vi "PQgetColumn.vi"(8 "error in":errorcluster, 10 "query":string, 11 "conn":u32) -> (0 "error out":errorcluster, 2 "Data":string[](array[string]), 3 "conn_out":u32)   [LabVIEW 2019, in "libpqutility.lvlib"]
uses:
  libpqutility.lvlib
  libpqlv/src/PQgetvalue.vi
  libpqlv/src/PQntuples.vi
  libpqlv/libpqlv.lvlib
panel:
  out "PQsendQuery":i32
  out "PQresultStatus":T1(ring)
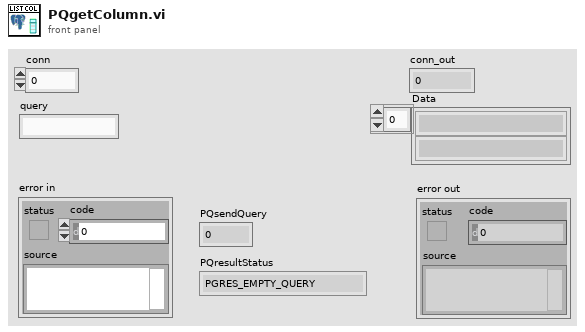
[diagram p1: front panel]
types:
  T1 = enum32{"PGRES_EMPTY_QUERY", "PGRES_COMMAND_OK", "PGRES_TUPLES_OK", "PGRES_COPY_OUT", "PGRES_COPY_IN", "PGRES_BAD_RESPONSE", "PGRES_NONFATAL_ERROR", "PGRES_FATAL_ERROR"}
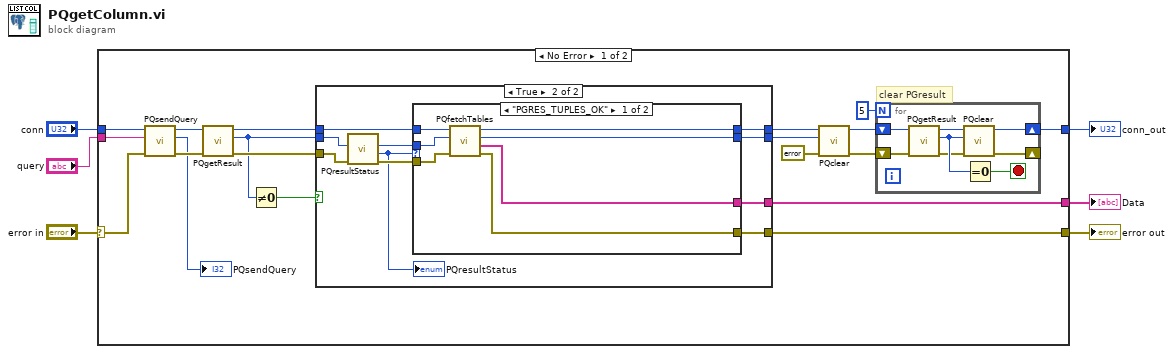
[diagram p0: block diagram]
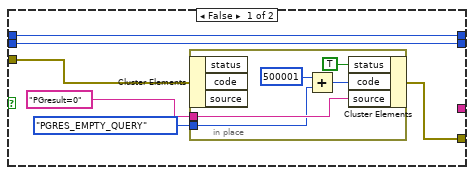
[diagram p2: hidden frame]
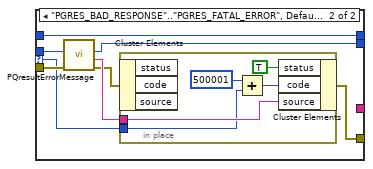
[diagram p3: hidden frame]
diagram:
  n1 = case shown="No Error" "error in" {
    selector: "error in" -> [w16 w76]
    tunnel: "conn" -> [w17 w75]
    tunnel: [w18 w76] -> w5
    tunnel: [w9 w75] -> w3
    tunnel: [w15 _] -> w2
    tunnel: "query" -> [w10 _]
    frame No Error {
      # "clear PGresult"
      n2 = call "PQsendQuery.vi"("error in (no error)"=w16, "query"=w10, "conn"=w17) -> ("error out"=w25:errorcluster, "PQsendQuery"=→"PQsendQuery":i32, "conn_out"=w14:u32)  [unwired: 6 in]
      n3 = call "PQgetResult.vi"("error in (no error)"=w25, "conn"=w14) -> ("error out"=w24:errorcluster, "PGresult"=w23:u32, "conn_out"=w13:u32)  [unwired: 7 in]
      n4 = Not Equal To 0?(x=w23) -> (x != 0?=w22:bool)
      n5 = case shown="True" w22 {
        tunnel: w24 -> [w28 w46]
        tunnel: w13 -> [w30 w45]
        tunnel: [_ w43] -> w15
        tunnel: [w27 w42] -> w18
        tunnel: w23 -> [w31 w41]
        tunnel: [w31 w39] -> w19
        tunnel: [w30 w37] -> w12
        frame False {
          n6 = in-place {
            in-place-border: "PGresult=0" ("source") -> [w36]
            in-place-border: T1."PGRES_EMPTY_QUERY" ("PQresultStatus") -> [w33]
            n7 = in-place-cluster #1(w28) -> ()  [unwired: 3 out]
            n8 = Add(x=u32 500001, y=w33) -> (x+y=w32:u32)
            n9 = in-place-cluster #1("status"=TRUE, "code"=w32, "source"=w36) -> (w27:errorcluster)
          }
        }
        frame True {
          n10 = call "PQresultStatus.vi"("error in (no error)"=w46, "res"=w41) -> ("error out"=w44:errorcluster, "PQresultStatus"=w40:T1, "res out"=w38:u32)  [unwired: 7 in]
          "PQresultStatus" <- w40
          n11 = case shown="\"PGRES_TUPLES_OK\"" w40 {
            selector: w40 -> [_ w57]
            tunnel: w38 -> [w52 w59]
            tunnel: w44 -> [w53 w61]
            tunnel: w45 -> [w51 w60]
            tunnel: [w50 _] -> w43
            tunnel: [w47 w55] -> w42
            tunnel: [w49 w58] -> w39
            tunnel: [w48 w60] -> w37
            frame "PGRES_TUPLES_OK" {
              n12 = call "PQfetchTables.vi"("error in"=w53, "res"=w52, "conn"=w51) -> ("error out"=w47:errorcluster, "Data"=w50:string[], "res_out"=w49:u32, "conn_out"=w48:u32)  [unwired: 3 in, 2 out]
            }
            frame "PGRES_BAD_RESPONSE".."PGRES_FATAL_ERROR", Default {
              n13 = call "PQresultErrorMessage.vi"("error in (no error)"=w61, "res"=w59) -> ("error out"=w54:errorcluster, "PQresultErrorMessage"=w56:string, "res out"=w58:u32)  [unwired: 7 in]
              n14 = in-place {
                in-place-border: w56 -> [w66]
                in-place-border: w57 -> [w63]
                n15 = in-place-cluster #2(w54) -> ()  [unwired: 3 out]
                n16 = Add(x=u32 500001, y=w63) -> (x+y=w62:u32)
                n17 = in-place-cluster #2("status"=TRUE, "code"=w62, "source"=w66) -> (w55:errorcluster)
              }
            }
          }
        }
      }
      n18 = call "PQclear.vi"("error in (no error)"=errorcluster {"status"=FALSE, "code"=0, "source"=""}, "res"=w19, "conn"=w12) -> ("error out"=w8:errorcluster, "conn_out"=w11:u32)  [unwired: 7 in]
      n19 = for {
        N: 5 -> [_]
        shift-right: [w70] -> w9
        shift-left: w11 -> [w71]
        shift-right: [w67] -> _
        shift-left: w8 -> [w69]
        stop <- w73 stop-if-true
        n20 = call "PQgetResult.vi"("error in (no error)"=w69, "conn"=w71) -> ("error out"=w68:errorcluster, "PGresult"=w72:u32, "conn_out"=w74:u32)  [unwired: 7 in]
        n21 = call "PQclear.vi"("error in (no error)"=w68, "res"=w72, "conn"=w74) -> ("error out"=w67:errorcluster, "conn_out"=w70:u32)  [unwired: 7 in]
        n22 = Equal To 0?(x=w72) -> (x = 0?=w73:bool)
      }
    }
    frame Error {
    }
  }
  "conn_out" <- w3
  "error out" <- w5
  "Data" <- w2
